vi "Read rect.vi"(8 "error in (no error)":errorcluster, 11 "FSM.Label in":refnum<class "FSM.Label.lvclass">) -> (0 "error out":errorcluster, 2 "rect":T1, 3 "FSM.Label out":refnum<class "FSM.Label.lvclass">)   [LabVIEW 2020, in "FSM.Label.lvclass"]
uses:
  FSM.Label.lvclass
  FSM.Label.lvclass/FSM.Label.ctl
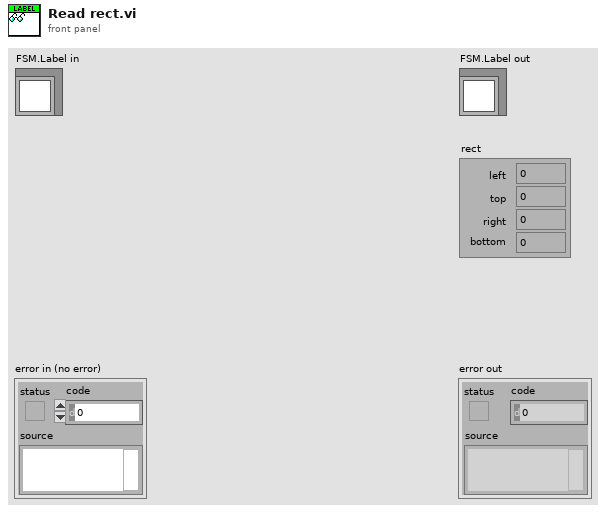
[diagram p1: front panel]
types:
  T1 = cluster{"left":i16, "top":i16, "right":i16, "bottom":i16}
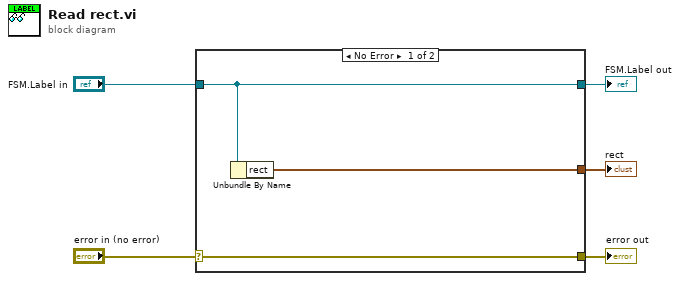
[diagram p0: block diagram]
diagram:
  n1 = case shown="No Error" "error in (no error)" {
    selector: "error in (no error)" -> [w8 w9]
    tunnel: [w8 w9] -> w4
    tunnel: [w7 w10] -> w2
    tunnel: "FSM.Label in" -> [w7 w10]
    tunnel: [w6 _] -> w1
    frame No Error {
      n2 = Unbundle By Name(w7) -> ("rect"=w6:T1)
    }
    frame Error {
    }
  }
  "error out" <- w4
  "FSM.Label out" <- w2
  "rect" <- w1
